vi "Table, Show All Columns.vi"(8 "error in":errorcluster, 11 "Tbl Refnum":refnum<vi>) -> (0 "error out":errorcluster, 3 "Tbl Refnum out":refnum<vi>)   [LabVIEW 2010]
doc: "Shows all table columns plus an empty column.\nSince all columns are displayed, the horizontal scrollbar is hidden."
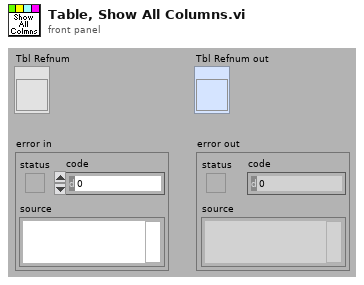
[diagram p1: front panel]
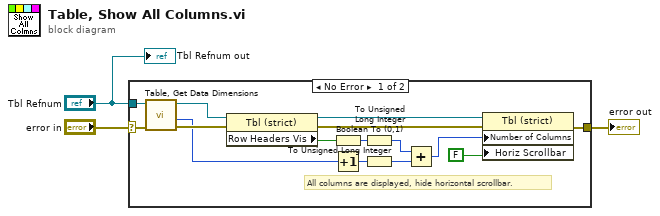
[diagram p0: block diagram]
diagram:
  n1 = case shown="No Error" "error in" {
    selector: "error in" -> [w15 w19]
    tunnel: [w11 w19] -> w3
    tunnel: "Tbl Refnum" -> [w16 _]
    frame No Error {
      # "All columns are displayed, hide horizontal scrollbar."
      n2 = call "Table, Get Data Dimensions.vi"("error in"=w15, "Tbl Refnum"=w16) -> ("error out"=w18:errorcluster, "col_n"=w4:i32, "Tbl Refnum out"=w17:refnum<vi>)  [unwired: 6 in, 1 out]
      n3 = property class="Tbl (strict)"(reference=w17, error in=w18) -> (reference out=w9:refnum<vi>, error out=w12:errorcluster, "Row Headers Vis"=w14:bool)
      n4 = Boolean To (0,1)(Boolean=w14) -> (0, 1=w7:i16)
      n5 = Increment(x=w4) -> (x+1=w13:i32)
      n6 = To Unsigned Long Integer(number=w7) -> (unsigned 32bit integer=w6:u32)
      n7 = To Unsigned Long Integer(number=w13) -> (unsigned 32bit integer=w8:u32)
      n8 = Add(x=w6, y=w8) -> (x+y=w10:u32)
      n9 = property class="Tbl (strict)"(reference=w9, error in=w12, "Number of Columns"=w10, "Horiz Scrollbar"=FALSE) -> (error out=w11:errorcluster)  [unwired: 1 out]
    }
    frame Error {
    }
  }
  "error out" <- w3
  "Tbl Refnum out" <- "Tbl Refnum"
